vi "running ini.vi"(0 "running in":bool, 1 "Action":T1, 2 "Ini file path":path) -> (4 "running out":bool)   [LabVIEW 2012]
uses:
  file/file action.ctl
  DAC project/Calibration and Function folders.ctl
  <vilib>/Utility/config.llb/Write Key (Boolean).vi
  <vilib>/Utility/config.llb/Read Key (Boolean).vi
  <vilib>/Utility/config.llb/NI_LVConfig.lvlib
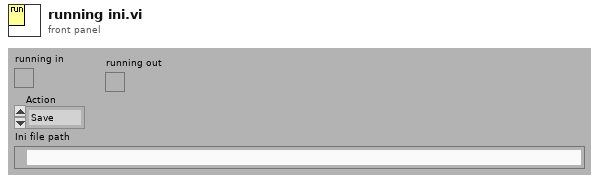
[diagram p1: front panel]
types:
  T1 = typedef "file action.ctl" = enum16{"Save", "Open"}
  T2 = typedef "Calibration and Function folders.ctl" = enum16{"Sensors", "Functions", "Config File", "UserAppFolder"}
  T3 = typedef "NI_LVConfig.lvlib/Config Data RefNum.ctl" = refnum<k1>
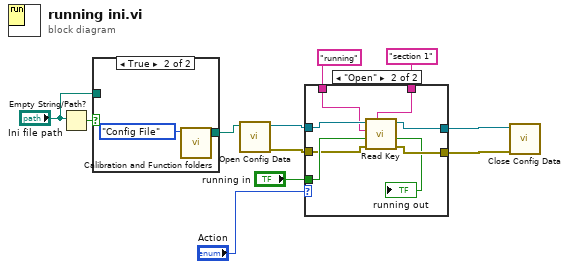
[diagram p0: block diagram]
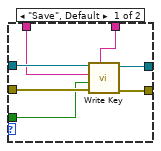
[diagram p3: hidden frame]
diagram:
  n1 = Empty String/Path?(string/path="Ini file path") -> (empty?=w2:bool)
  n2 = case shown="True" w2 {
    tunnel: [w12 w13] -> w11
    tunnel: "Ini file path" -> [w12 _]
    frame False {
    }
    frame True {
      n3 = call "Calibration and Function folders.vi"("Folder"=Calibration_and_Function_folders."Config File") -> ("Selected Folder"=w13:path)  [unwired: 10 in]
    }
  }
  n4 = call <vilib>:"Open Config Data.vi"("configuration file path"=w11) -> ("error out"=w10:errorcluster, "refnum"=w8:T3)  [unwired: 8 in, 1 out]
  n5 = case shown="\"Open\"" "Action" {
    tunnel: w10 -> [w21 w24]
    tunnel: [w20 w23] -> w9
    tunnel: w8 -> [w19 w29]
    tunnel: [w18 w28] -> w7
    tunnel: "section 1" ("section") -> [w17 w27]
    tunnel: "running" ("key") -> [w16 w26]
    tunnel: "running in" -> [w15 w25]
    frame "Save", Default {
      n6 = call-poly <vilib>:"Write Key.vi"("section"=w17, "error in (no error)"=w21, "value"=w15, "key"=w16, "refnum"=w19) -> ("error out"=w20:errorcluster, "refnum out"=w18:T3)  [unwired: 4 in, 1 out]
    }
    frame "Open" {
      n7 = call-poly <vilib>:"Read Key.vi"("section"=w27, "error in (no error)"=w24, "default value"=w25, "key"=w26, "refnum"=w29) -> ("error out"=w23:errorcluster, "value"=→"running out":bool, "refnum out"=w28:T3)  [unwired: 3 in, 1 out]
    }
  }
  n8 = call <vilib>:"Close Config Data.vi"("error in (no error)"=w9, "refnum"=w7) -> ()  [unwired: 8 in, 2 out]
